vi "ExpTimeConversion.vi"(8 "PrevExpTime_ms":i32, 9 "PrevActualTime_ms":i32, 11 "time stamp":timestamp) -> (0 "ExpTime_ms":i32, 1 "ActualTime_ms":i32, 2 "ActualTimeString":string="0", 3 "ActualDateString":string="0")   [LabVIEW 2020]
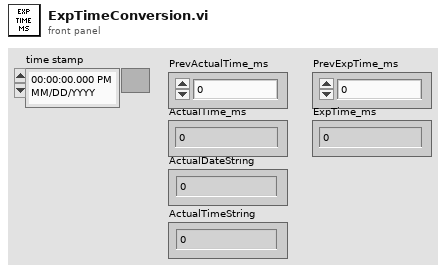
[diagram p1: front panel]
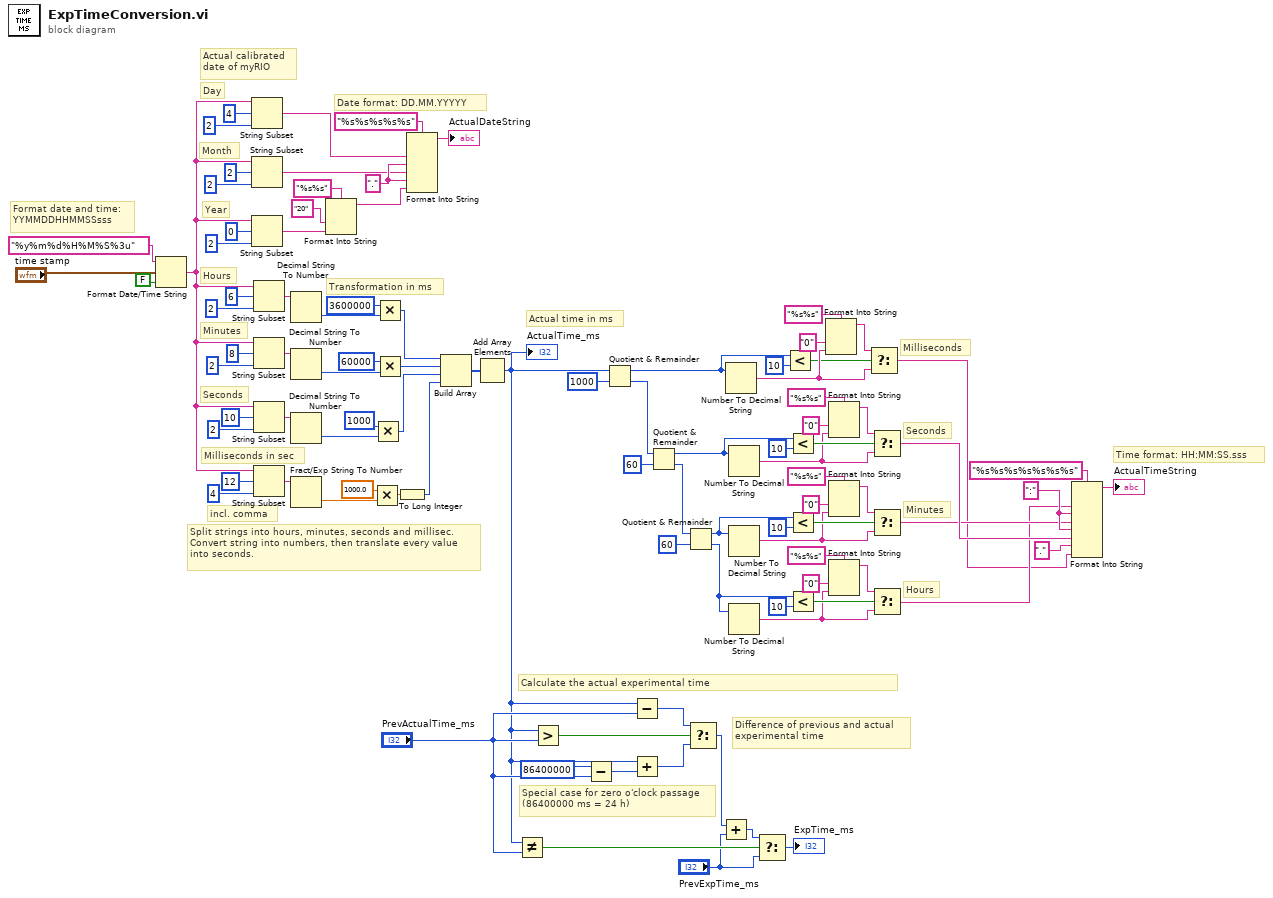
[diagram p0: block diagram]
diagram:
  w41 = "." ("input 4")
  w69 = ":"
  # "Special case for zero o'clock passage\n(86400000 ms = 24 h)"
  # "Difference of previous and actual\nexperimental time"
  # "Calculate the actual experimental time"
  # "Milliseconds"
  # "incl. comma"
  # "Transformation in ms"
  # "Milliseconds in sec"
  # "Seconds"
  # "Minutes"
  # "Hours"
  # "Format date and time: \nYYMMDDHHMMSSsss"
  # "Date format: DD.MM.YYYYY"
  # "Time format: HH:MM:SS.sss"
  # "Hours"
  # "Minutes"
  # "Seconds"
  # "Actual time in ms"
  # "Day"
  # "Month"
  # "Year"
  # "Actual calibrated \ndate of myRIO"
  # "Split strings into hours, minutes, seconds and millisec. \nConvert string into numbers, then translate every value\ninto seconds."
  n1 = Format Date/Time String(time format string (%c)="%y%m%d%H%M%S%3u", seconds (now)="time stamp", UTC format=FALSE ("want seconds? (F)")) -> (date/time string=w32:string)
  n2 = String Subset(string=w32, offset (0)=4, length (rest)=2 ("length (rest)")) -> (substring=w38:string)
  n3 = String Subset(string=w32, offset (0)=2, length (rest)=2 ("length (rest)")) -> (substring=w39:string)
  n4 = String Subset(string=w32, offset (0)=0, length (rest)=2 ("length (rest)")) -> (substring=w37:string)
  n5 = String Subset(string=w32, offset (0)=6, length (rest)=2 ("length (rest)")) -> (substring=w98:string)
  n6 = String Subset(string=w32, offset (0)=8, length (rest)=2 ("length (rest)")) -> (substring=w91:string)
  n7 = String Subset(string=w32, offset (0)=10, length (rest)=2 ("length (rest)")) -> (substring=w90:string)
  n8 = String Subset(string=w32, offset (0)=12, length (rest)=4 ("length (rest)")) -> (substring=w35:string)
  n9 = Decimal String To Number(string=w98) -> (number=w89:i32)  [unwired: 2 in, 1 out]
  n10 = Decimal String To Number(string=w91) -> (number=w87:i32)  [unwired: 2 in, 1 out]
  n11 = Decimal String To Number(string=w90) -> (number=w30:i32)  [unwired: 2 in, 1 out]
  n12 = Fract/Exp String To Number(string=w35) -> (number=w27:dbl)  [unwired: 3 in, 1 out]
  n13 = Format Into String(format string="%s%s", "20" ("input 1"), w37) -> (resulting string=w36:string)  [unwired: 2 in, 1 out]
  n14 = Multiply(x=1000.0, y=w27) -> (x*y=w26:dbl)
  n15 = Multiply(x=1000, y=w30) -> (x*y=w29:i32)
  n16 = Multiply(x=3600000, y=w89) -> (x*y=w85:i32)
  n17 = Multiply(x=60000, y=w87) -> (x*y=w84:i32)
  n18 = To Long Integer(number=w26) -> (32bit integer=w25:i32)
  n19 = Format Into String(format string="%s%s%s%s%s", w38, w41, w39, w41, w36) -> (resulting string=→"ActualDateString":string)  [unwired: 2 in, 1 out]
  n20 = Build Array(w85, w84, w29, w25) -> (w83:i32[])
  n21 = Add Array Elements(numeric array=w83) -> (sum=w2:i32)
  "ActualTime_ms" <- w2
  n22 = Not Equal?(x=w2, y="PrevActualTime_ms") -> (x != y?=w13:bool)
  n23 = Greater?(x=w2, y="PrevActualTime_ms") -> (0:w9:bool)
  n24 = Subtract(x=86400000, y="PrevActualTime_ms") -> (x-y=w3:i32)
  n25 = Quotient & Remainder(x=w2, y=1000) -> (x-y*floor(x/y)=w23:i32, floor(x/y)=w14:i32)
  n26 = Subtract(x=w2, y="PrevActualTime_ms") -> (x-y=w7:i32)
  n27 = Add(x=w2, y=w3) -> (x+y=w4:i32)
  n28 = Quotient & Remainder(x=w14, y=60) -> (x-y*floor(x/y)=w60:i32, floor(x/y)=w71:i32)
  n29 = Quotient & Remainder(x=w71, y=60) -> (x-y*floor(x/y)=w51:i32, floor(x/y)=w43:i32)
  n30 = Select(t=w7, s=w9, f=w4) -> (s? t:f=w8:i32)
  n31 = Add(x=w8, y="PrevExpTime_ms") -> (x+y=w12:i32)
  n32 = Number To Decimal String(number=w23) -> (decimal integer string=w22:string)  [unwired: 1 in]
  n33 = Number To Decimal String(number=w60) -> (decimal integer string=w61:string)  [unwired: 1 in]
  n34 = Number To Decimal String(number=w51) -> (decimal integer string=w52:string)  [unwired: 1 in]
  n35 = Number To Decimal String(number=w43) -> (decimal integer string=w45:string)  [unwired: 1 in]
  n36 = Select(t=w12, s=w13, f="PrevExpTime_ms") -> (s? t:f=→"ExpTime_ms":i32)
  n37 = Less?(x=w23, y=10) -> (x < y?=w18:bool)
  n38 = Less?(x=w60, y=10) -> (x < y?=w66:bool)
  n39 = Less?(x=w51, y=10) -> (x < y?=w55:bool)
  n40 = Less?(x=w43, y=10) -> (x < y?=w49:bool)
  n41 = Format Into String(format string="%s%s", "0" ("input 1"), w22) -> (resulting string=w21:string)  [unwired: 2 in, 1 out]
  n42 = Format Into String(format string="%s%s", "0" ("input 1"), w61) -> (resulting string=w63:string)  [unwired: 2 in, 1 out]
  n43 = Format Into String(format string="%s%s", "0" ("input 1"), w52) -> (resulting string=w58:string)  [unwired: 2 in, 1 out]
  n44 = Format Into String(format string="%s%s", "0" ("input 1"), w45) -> (resulting string=w46:string)  [unwired: 2 in, 1 out]
  n45 = Select(t=w21, s=w18, f=w22) -> (s? t:f=w15:string)
  n46 = Select(t=w63, s=w66, f=w61) -> (s? t:f=w62:string)
  n47 = Select(t=w58, s=w55, f=w52) -> (s? t:f=w53:string)
  n48 = Select(t=w46, s=w49, f=w45) -> (s? t:f=w44:string)
  n49 = Format Into String(format string="%s%s%s%s%s%s%s", w44, w69, w53, w69, w62, ".", w15) -> (resulting string=→"ActualTimeString":string)  [unwired: 2 in, 1 out]
